vi "Generated Descriptors.vi"() -> (3 "Descriptor Strings":string[](array[string]))   [LabVIEW 2021, in "test_service_server.lvlib"]
uses:
  test_service_server.lvlib
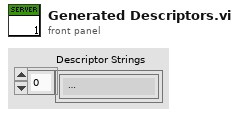
[diagram p1: front panel]
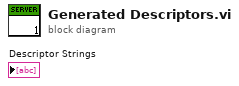
[diagram p0: block diagram]
diagram:
